vi "MH_WritePTUTag.vi"(4 "TagAuxData":string, 5 "TagValue":i64=80 format="%x", 6 "refnum":refnum<file>, 7 "error in":errorcluster, 8 "TagType":i32=80 format="%x", 9 "TagIndex":i32=80, 10 "identifierfull":string) -> (0 "error out":errorcluster)   [LabVIEW 2019]
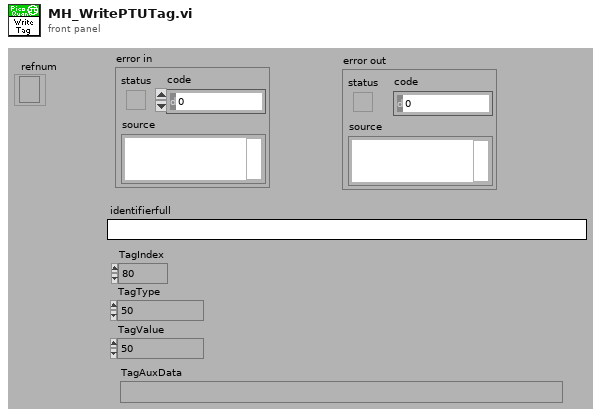
[diagram p1: front panel]
types:
  T1 = enum16{"big-endian, network order", "native, host order", "little-endian"}
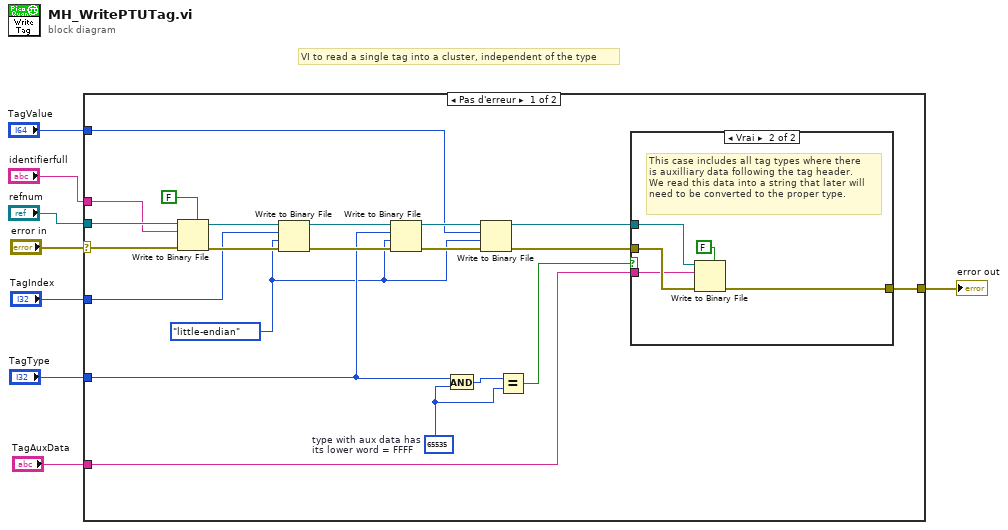
[diagram p0: block diagram]
diagram:
  # "VI to read a single tag into a cluster, independent of the type"
  n1 = case shown="Pas d'erreur" "error in" {
    selector: "error in" -> [w17 w36]
    tunnel: "refnum" -> [w19 _]
    tunnel: [w18 w36] -> w7
    tunnel: "identifierfull" -> [w16 _]
    tunnel: "TagIndex" -> [w13 _]
    tunnel: "TagType" -> [w11 _]
    tunnel: "TagValue" -> [w12 _]
    tunnel: "TagAuxData" -> [w15 _]
    frame No Error {
      w10 = T1."little-endian" ("ordre des octets (0 : big-Endian, network order)")
      w22 = 65535  # type with aux data has  its lower word = FFFF
      n2 = Write to Binary File(file (use dialog)=w19, data=w16, error in=w17, 5:FALSE ("ajouter une taille de tableau ou de chaîne ? (V)")) -> (refnum out=w25:refnum<file>, error out=w20:errorcluster)  [unwired: 2 in, 1 out]
      n3 = Write to Binary File(file (use dialog)=w25, data=w13, error in=w20, 9:w10) -> (refnum out=w27:refnum<file>, error out=w26:errorcluster)  [unwired: 2 in, 1 out]
      n4 = Write to Binary File(file (use dialog)=w27, data=w11, error in=w26, 9:w10) -> (refnum out=w28:refnum<file>, error out=w29:errorcluster)  [unwired: 2 in, 1 out]
      n5 = And(x=w11, y=w22) -> (x .and. y?=w23:i32)
      n6 = Write to Binary File(file (use dialog)=w28, data=w12, error in=w29, 9:w10) -> (refnum out=w9:refnum<file>, error out=w21:errorcluster)  [unwired: 2 in, 1 out]
      n7 = Equal?(x=w23, y=w22) -> (x = y?=w24:bool)
      n8 = case shown="Vrai" w24 {
        tunnel: w9 -> [_ w34]
        tunnel: w21 -> [w30 w35]
        tunnel: [w30 w33] -> w18
        tunnel: w15 -> [_ w32]
        frame False {
          # "This case includes all tag types that have NO \nauxilliary data. The corresponding string \nremains empty"
        }
        frame True {
          # "This case includes all tag types where there \nis auxilliary data following the tag header. \nWe read this data into a string that later will \nneed to be converted to the proper type."
          n9 = Write to Binary File(file (use dialog)=w34, data=w32, error in=w35, 5:FALSE ("ajouter une taille de tableau ou de chaîne ? (V)")) -> (error out=w33:errorcluster)  [unwired: 2 in, 2 out]
        }
      }
    }
    frame Error {
      # "Do nothing when there is already an error."
    }
  }
  "error out" <- w7
